vi "FindLaserDot.vi"(11 "Image Input":T1=refnum) -> (0 "Y Location":i32=143, 1 "X Location":i32=1050, 2 "Max Pixel Value":i32=100, 3 "Object Aquired":bool=TRUE)   [LabVIEW 2015]
uses:
  <vilib>/vision/Image Controls.llb/IMAQ Image.ctl
panel:
  in  "Pixel Brightness Threshold":i32=250
  out "image display":T1(plugin-control)
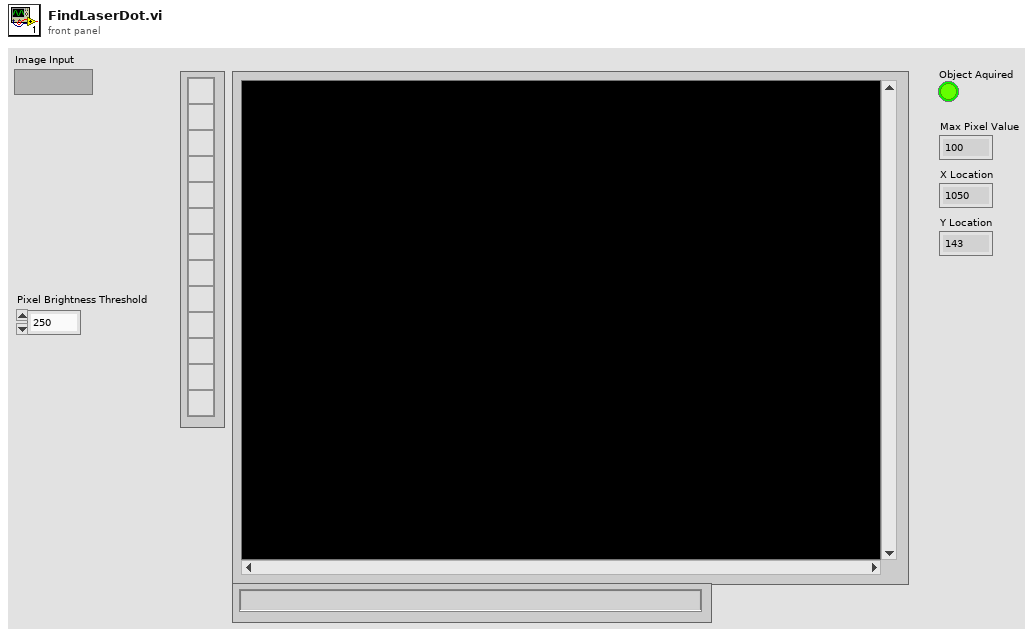
[diagram p1: front panel]
types:
  T1 = typedef "IMAQ Image.ctl" = refnum<image>
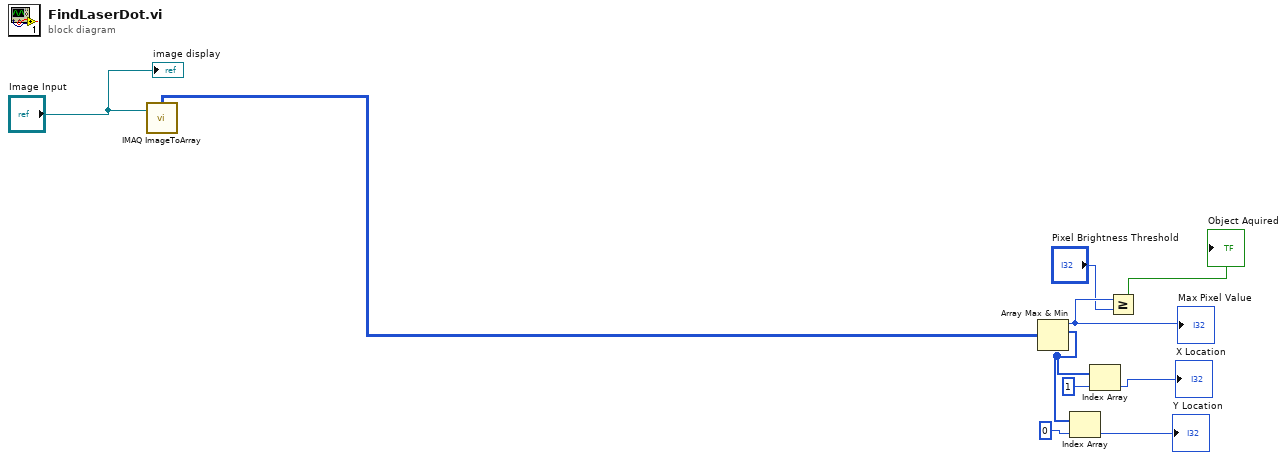
[diagram p0: block diagram]
diagram:
  n1 = call "IMAQ ImageToArray"("Image"="Image Input") -> ("Image Pixels (U8)"=w6:u8[][])  [unwired: 2 in, 5 out]
  n2 = Array Max & Min(array=w6) -> (max value=w9:u8, max index (indices)=w5:i32[])  [unwired: 2 out]
  "Max Pixel Value" <- w9
  n3 = Index Array(array=w5, index=0) -> (element=→"Y Location":i32)
  n4 = Index Array(array=w5, index=1) -> (element=→"X Location":i32)
  n5 = Greater Or Equal?(x=w9, y="Pixel Brightness Threshold") -> (x >= y?=→"Object Aquired":bool)
  "image display" <- "Image Input"
